vi "Main_fsTA.vi"() -> ()   [LabVIEW 2025]
uses:
  <vilib>/Math Plots/3D Math Plots/3D Surface/3D Surface XCtrl/3D Surface.xctl
  SubVI/TA_DATA.ctl
  <vilib>/Math Plots/3D Math Plots/3D Surface/3D Surface Datatype/Public/Plot Helper (Vector).vi
  <vilib>/Math Plots/3D Math Plots/3D Surface/3D Surface Datatype/3D Surface Datatype.lvclass
panel:
  out "TA Data":T1
  in  "Tab Control":T2(tab)
  in  "Delay Time":T3(ring)
  out "Generated Delay Time (ps)":dbl[](array[numeric])
  out "Number (Delay Time)":i32
  in  "Input for Generating Delay Time":T4(tab)
  in  "Step (ps)":dbl[](array[numeric])=[0.5, 0.05, 0.1, 0.5, 1.0, 2.0, 10.0, 100.0]
  in  "Time Range (ps)":dbl[](array[numeric])=[-10.0, -1.0, 1.0, 5.0, 20.0, 100.0, 500.0, 1000.0, 8000.0]
  in  "Linear \nTime Range (ps)":dbl[](array[numeric])=[-10.0, -1.0, 1.0]
  in  "Exponential \nTime Range (ps)":dbl[](array[numeric])=[1.0, 10.0, 100.0, 1000.0, 10000.0]
  in  "Linear\nStep (ps)":dbl[](array[numeric])=[0.5, 0.05]
  in  "Exponential\nNumber of Steps":dbl[](array[numeric])=[100.0, 100.0, 100.0, 100.0]
  in  "Random\nNumber of Steps":dbl[](array[numeric])=[200.0, 200.0, 100.0, 50.0]
  in  "Random \nTime Range (ps)":dbl[](array[numeric])=[1.0, 10.0, 100.0, 1000.0, 8000.0]
  in  "Linear\nStep (ps) 2":dbl[](array[numeric])=[0.5, 0.05]
  in  "Linear \nTime Range (ps) 2":dbl[](array[numeric])=[-10.0, -1.0, 1.0]
  in  "File Path 2":path=path "/Users/tm/Desktop/fs-TA/Data/demo_fsta2.dat"
  in  "Excitation Wavelength":string="800nm"
  in  "Sample":string="sample"
  in  "Solvent":string="solvent"
  in  "Excitation Energy":string="1uj"
  in  "Comments":string="XXXX"
  in  "_scan/_average":enum16{"_scan", "_average"}(ring)=enum."_average"
  in  "Current Scan":i16=1
  in  "Data Extension (.dat; .csv)":string=".dat"
  in  "Data Folder":path
  out "Filepath":path
  out "Kinetics":cluster{"Array":dbl[], "Array 2":dbl[]}[](graph)
  out "Raw TA":dbl[][](array[numeric]) format="%#_8g"
  in  "File Path":path=path "/Users/tm/Desktop/fs-TA/Data/demo_fsta.dat"
  out "Size (Raw TA)":i32[](array[numeric])
  in  "Wavelength (nm)":dbl[](array[numeric])
  in  "Update\nSelected\nWavelength":bool
  out "Spectra":cluster{"Array":dbl[], "Array 2":dbl[]}[](graph)
  in  "Time (ps)":dbl[](array[numeric])
  in  "Apply\nSelected\nDelay Time":bool
  out "TA 3D Surface":refnum<class "3D Plot Datatype.lvclass">[](xcontrol)
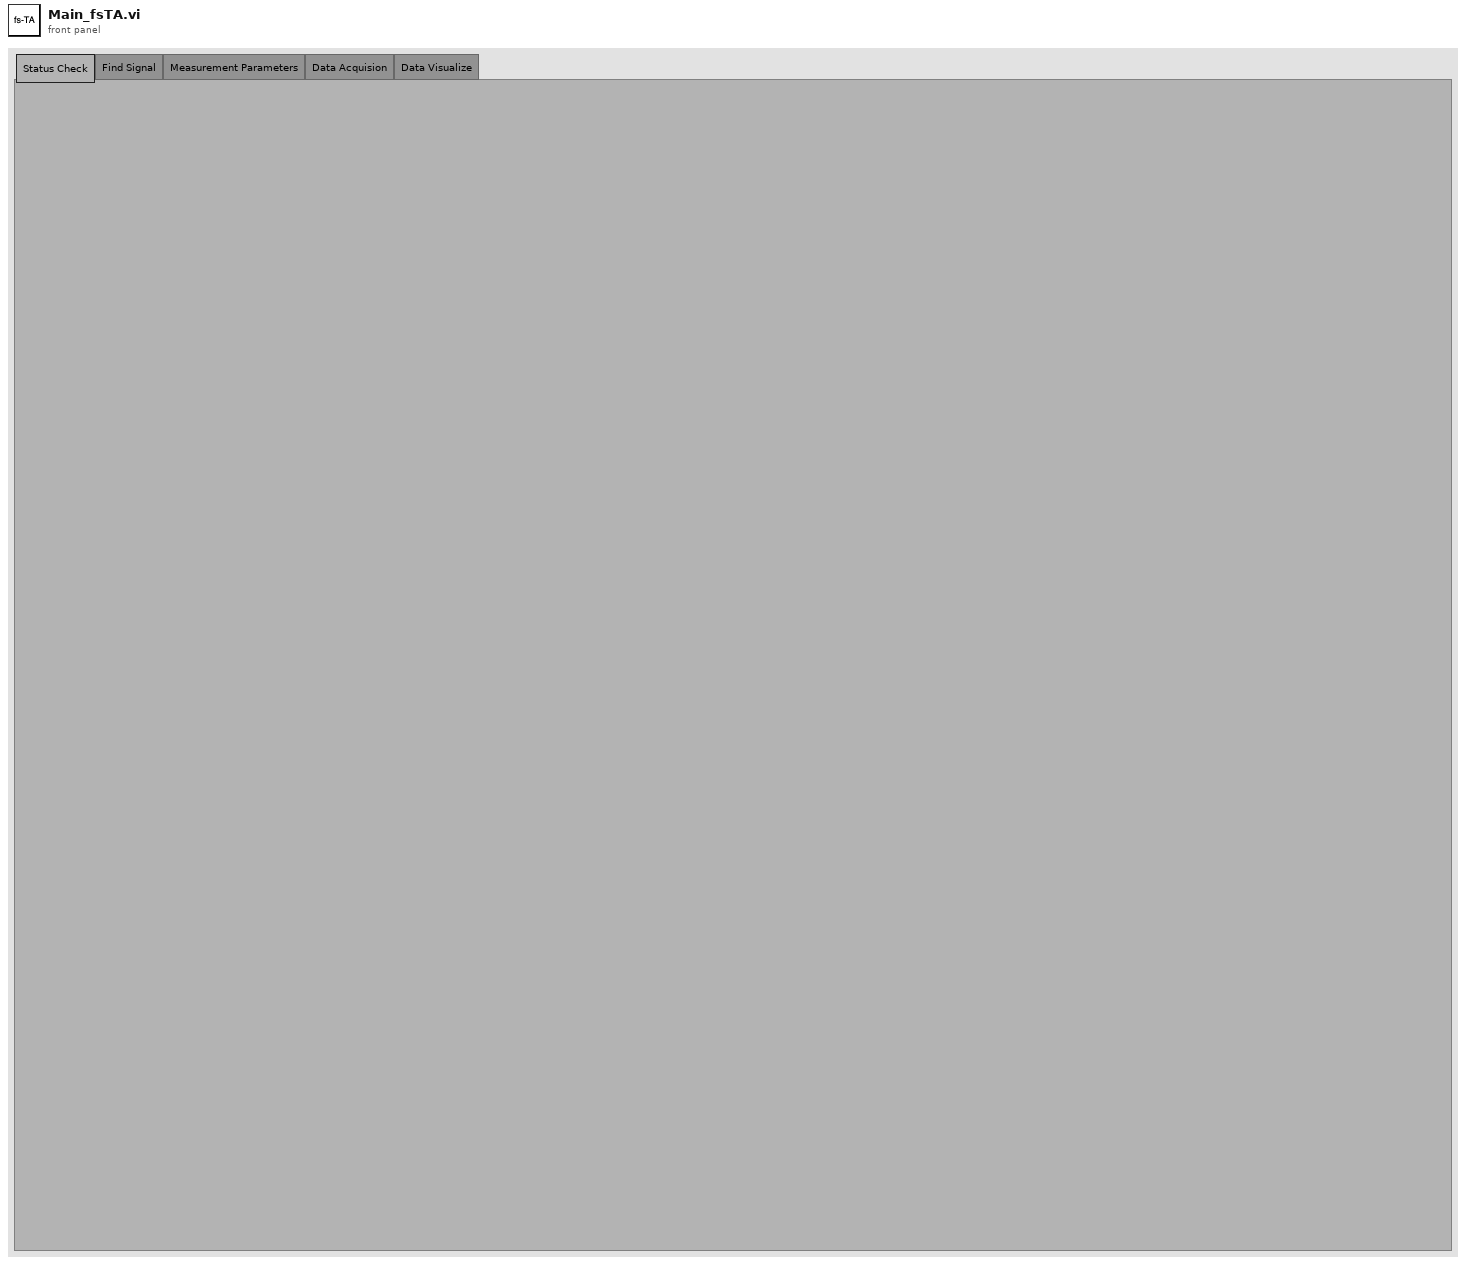
[diagram p1: front panel]
types:
  T1 = typedef "TA_DATA.ctl" = cluster{"DeltaA (mOD)":dbl[][], "Wavelength (nm)":dbl[], "Time (ps)":dbl[], "Size of DeltaA":i32[], "Size of Wavelength":i32, "Size of Time":i32}
  T2 = enum32{"Status Check", "Find Signal", "Measurement Parameters", "Data Acquision", "Data Visualize"}
  T3 = enum16{"Linear", "Linear+Exponential", "Linear+Random", "Load from File"}
  T4 = enum32{"Linear", "Linear+Exponential", "Linear+Random", "Load from File"}
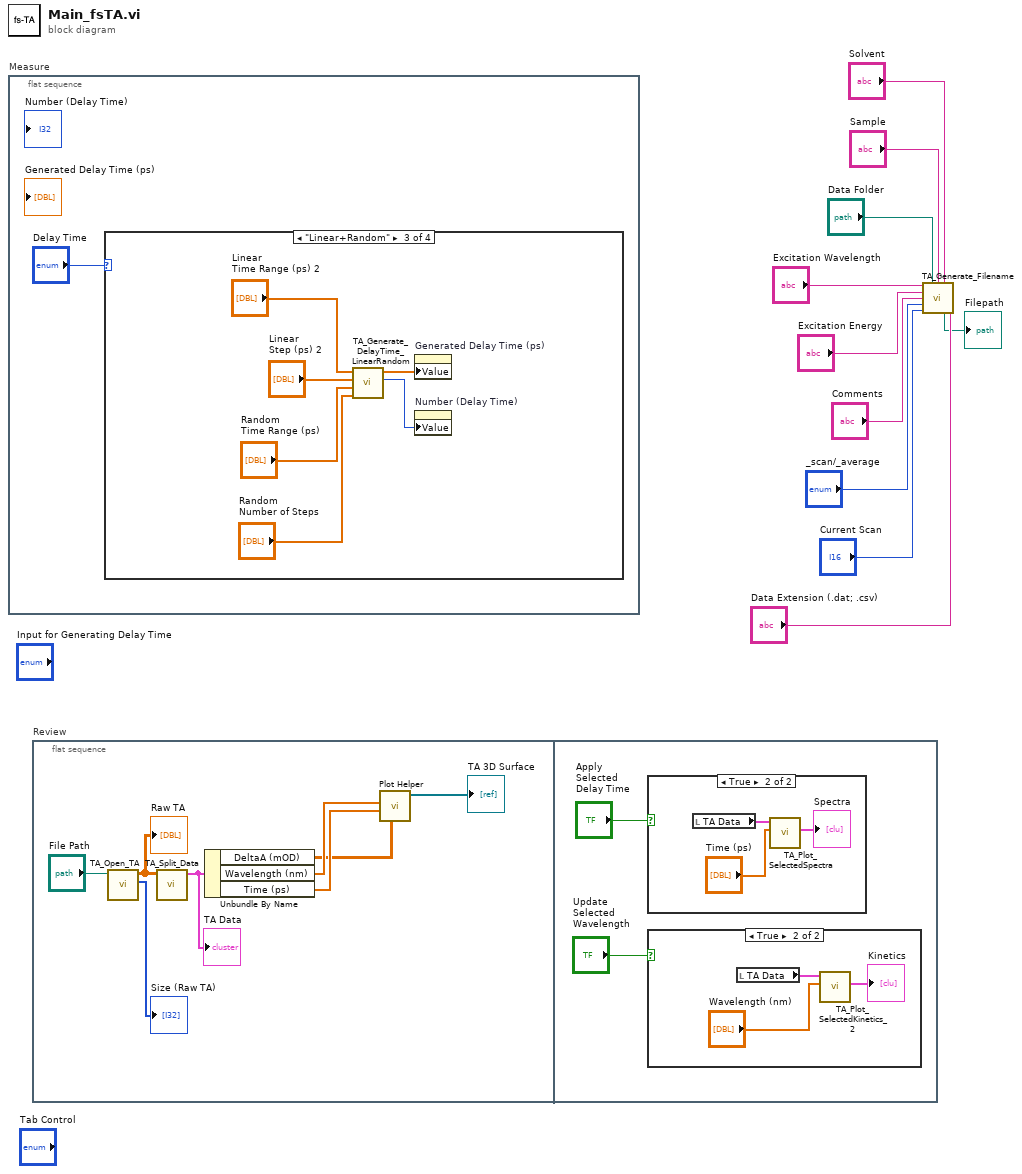
[diagram p0: block diagram]
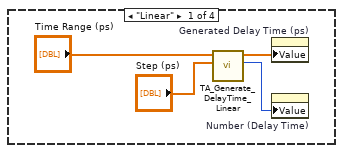
[diagram p4: hidden frame]
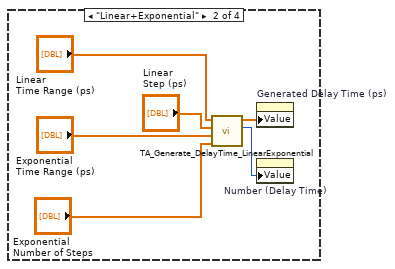
[diagram p5: hidden frame]
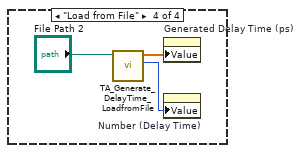
[diagram p6: hidden frame]
diagram:
  n1 = flat-sequence "Measure" {
    frame #0 {
      n2 = case shown="\"Linear+Random\"" "Delay Time" {
        frame "Linear" {
          n3 = call "TA_Generate_DelayTime_Linear.vi"("Step (ps)"="Step (ps)", "Time Range (ps)"="Time Range (ps)") -> ("Number (Delay Time)"=w12:i32, "Generated Delay Time (ps)"=w13:dbl[])  [unwired: 8 in]
          n4 = property on="Generated Delay Time (ps)" class="Arr (strict)"("Value"=w13) -> ()  [unwired: 2 in, 2 out]
          n5 = property on="Number (Delay Time)" class="DigNum (strict)"("Value"=w12) -> ()  [unwired: 2 in, 2 out]
        }
        frame "Linear+Exponential" {
          n6 = call "TA_Generate_DelayTime_LinearExponential.vi"("Exponential\nNumber of Steps"="Exponential\nNumber of Steps", "Exponential \nTime Range (ps)"="Exponential \nTime Range (ps)", "Linear\nStep (ps)"="Linear\nStep (ps)", "Linear \nTime Range (ps)"="Linear \nTime Range (ps)") -> ("Number (Delay Time)"=w16:i32, "Generated Delay Time (ps)"=w17:dbl[])  [unwired: 6 in]
          n7 = property on="Generated Delay Time (ps)" class="Arr (strict)"("Value"=w17) -> ()  [unwired: 2 in, 2 out]
          n8 = property on="Number (Delay Time)" class="DigNum (strict)"("Value"=w16) -> ()  [unwired: 2 in, 2 out]
        }
        frame "Linear+Random" {
          n9 = call "TA_Generate_DelayTime_LinearRandom.vi"("Random\nNumber of Steps"="Random\nNumber of Steps", "Random \nTime Range (ps)"="Random \nTime Range (ps)", "Linear\nStep (ps)"="Linear\nStep (ps) 2", "Linear \nTime Range (ps)"="Linear \nTime Range (ps) 2") -> ("Number (Delay Time)"=w22:i32, "Generated Delay Time (ps)"=w23:dbl[])  [unwired: 6 in]
          n10 = property on="Generated Delay Time (ps)" class="Arr (strict)"("Value"=w23) -> ()  [unwired: 2 in, 2 out]
          n11 = property on="Number (Delay Time)" class="DigNum (strict)"("Value"=w22) -> ()  [unwired: 2 in, 2 out]
        }
        frame "Load from File" {
          n12 = call "TA_Generate_DelayTime_LoadfromFile.vi"("File Path"="File Path 2") -> ("Number (Delay Time)"=w28:i32, "Generated Delay Time (ps)"=w29:dbl[])  [unwired: 9 in]
          n13 = property on="Generated Delay Time (ps)" class="Arr (strict)"("Value"=w29) -> ()  [unwired: 2 in, 2 out]
          n14 = property on="Number (Delay Time)" class="DigNum (strict)"("Value"=w28) -> ()  [unwired: 2 in, 2 out]
        }
      }
    }
  }
  n15 = flat-sequence "Review" {
    frame #0 {
      n16 = call "TA_Open_TA.vi"("Path"="File Path") -> ("Size (Raw TA)"=→"Size (Raw TA)":i32[], "Raw TA"=w31:dbl[][])  [unwired: 9 in]
      "Raw TA" <- w31
      n17 = call "TA_Split_Data.vi"("Raw TA"=w31) -> ("TA Data"=w32:T1)  [unwired: 10 in]
      "TA Data" <- w32
      n18 = Unbundle By Name(w32) -> ("DeltaA (mOD)"=w33:dbl[][], "Wavelength (nm)"=w35:dbl[], "Time (ps)"=w34:dbl[])
      n19 = call-poly <vilib>:"Plot Helper.vi"("z matrix"=w33, "y vector"=w34, "x vector"=w35) -> ("3D Plot lvclass Array out"=→"TA 3D Surface":refnum<class "3D Plot Datatype.lvclass">[])  [unwired: 3 in, 5 out]
    }
    frame #1 {
      n20 = case shown="True" "Apply\nSelected\nDelay Time" {
        frame False {
        }
        frame True {
          n21 = local read "TA Data"() -> (w43:T1)
          n22 = call "TA_Plot_SelectedSpectra.vi"("Selected Time (ps)"="Time (ps)", "TA Data"=w43) -> ("TA Selected Spectra"=→"Spectra":cluster{"Array":dbl[], "Array 2":dbl[]}[])  [unwired: 6 in, 1 out]
        }
      }
      n23 = case shown="True" "Update\nSelected\nWavelength" {
        frame False {
        }
        frame True {
          n24 = local read "TA Data"() -> (w44:T1)
          n25 = call "TA_Plot_SelectedKinetics_2.vi"("Selected\nWavelength (nm)"="Wavelength (nm)", "TA Data"=w44) -> ("TA Selected Kinetics"=→"Kinetics":cluster{"Array":dbl[], "Array 2":dbl[]}[])  [unwired: 6 in, 1 out]
        }
      }
    }
  }
  n26 = call "TA_Generate_Filename.vi"("Excitation Wavelength"="Excitation Wavelength", "Root Folder"="Data Folder", "Sample"="Sample", "Solvent"="Solvent", "Excitation Energy"="Excitation Energy", "Comments"="Comments", "_scan/_average"="_scan/_average", "Current Scan"="Current Scan", "Data Extension (.dat; .csv)"="Data Extension (.dat; .csv)") -> ("Filepath"=→"Filepath":path)  [unwired: 4 in, 2 out]
